vi "SCRAnalysis.vi"() -> ()   [LabVIEW 2013]
uses:
  <vilib>/Analysis/2dsp.llb/Decimate (single shot, DBL).vi
  <vilib>/Analysis/baseanly.llb/Real Dot Product.vi
  <vilib>/Utility/file.llb/Read From Spreadsheet File (DBL).vi
  <vilib>/Utility/file.llb/Read From Spreadsheet File (string).vi
  <vilib>/Utility/file.llb/Write To Spreadsheet File (DBL).vi
  <vilib>/measure/macond.llb/IIR Filter for 1 Chan.vi
  <vilib>/measure/maresamp.llb/Resample Waveform (single shot).vi
  <vilib>/Waveform/WDTFileIO.llb/Export Waveform To Spreadsheet File.vi
  <vilib>/Waveform/WDTFileIO.llb/ Write Waveform to File.vi
  <vilib>/Utility/file.llb/Write To Spreadsheet File (string).vi
  <vilib>/Analysis/NI_AALBase.lvlib
  <vilib>/Analysis/NI_AALPro.lvlib
  <vilib>/measure/NI_MAPro.lvlib
panel:
  out "subarray":string[][](array[string])
  out "raw data":dbl[][](array[numeric])
  in  "Tab Control":enum32{"Data Preprocessing", "SCR Analysis"}(tab)
  in  "Load Data":bool
  out "Cleaned Data":waveform(dbl)(graph)={"t0"=timestamp(0 s since 1904-01-01), "dt"=0.05, "Y"=[]}
  in  "Create Event Onset Files from Markers":bool caption="OK Button"
  in  "column containing SCR":i32=1
  in  "Start marker":string
  in  "Event markers of interest":string[](array[string])=["", "", "", "", "", "", "", "", "", "", "", ""]
  in  "Sample Rate (Hz)":dbl=20.0
  in  "Save Cleaned Data":bool
  in  "Apply New Settings":bool
  in  "New Sample Rate (Hz)":i32=25
  out "Raw Data":waveform(dbl)(graph)={"t0"=timestamp(0 s since 1904-01-01), "dt"=0.05, "Y"=[]}
  in  "Rank":i32=3 min=1
  in  "Filter?":bool
  in  "Median Filter?":bool
  in  "Resample Data":bool
  in  "IIR filter specifications":T1={"Topology"=enum."Butterworth", "Type"=enum."Bandpass", "Order"=1, "Lower Fc"=0.1, "Upper Fc"=5.0, "PB Ripple"=1.0, "SB Attenuation"=60.0} {"PB Ripple" format="%0.2f"; "SB Attenuation" format="%0.2f"; "Lower Fc" format="%0.2p"; "Upper Fc" format="%0.2p"}
  out "Event  Timepoints (in samples - first number in each row is number of events detected in the file)":i32[][](array[numeric])
  in  "column containing markers":i32=2
  out "start marker detected at row":i32
  in  "append text to start of each line":string
  in  "Timing file names":string
  in  "Timing file directory":path
  out "residual":dbl=0.00434139012463345
  in  "Event Offset (s)":dbl=-2.0
  in  "Save Coefficients":bool
  out "Basis Set":dbl[][](graph)
  out "Event-related responses":dbl[][](graph)
  out "All Regressors":dbl[][](graph)
  out "Data and Fitted Response":dbl[][](graph)
  in  "Number of Basis Functions":i32=8
  in  "Window Length (s)":dbl=12.0
  out "Coefficients (GLM parameter estimates)":dbl[](array[numeric])
  in  "recalculate":bool
  in  "Save Response Data":bool
  in  "decimating factor":i32=1
  in  "Basis Set":u16(ring)=1 items=["Fourier", "Tents", "Blocks"]
  in  "append to existing files?":bool
  # "Data Preprocessing"
  # "SCR Analysis"
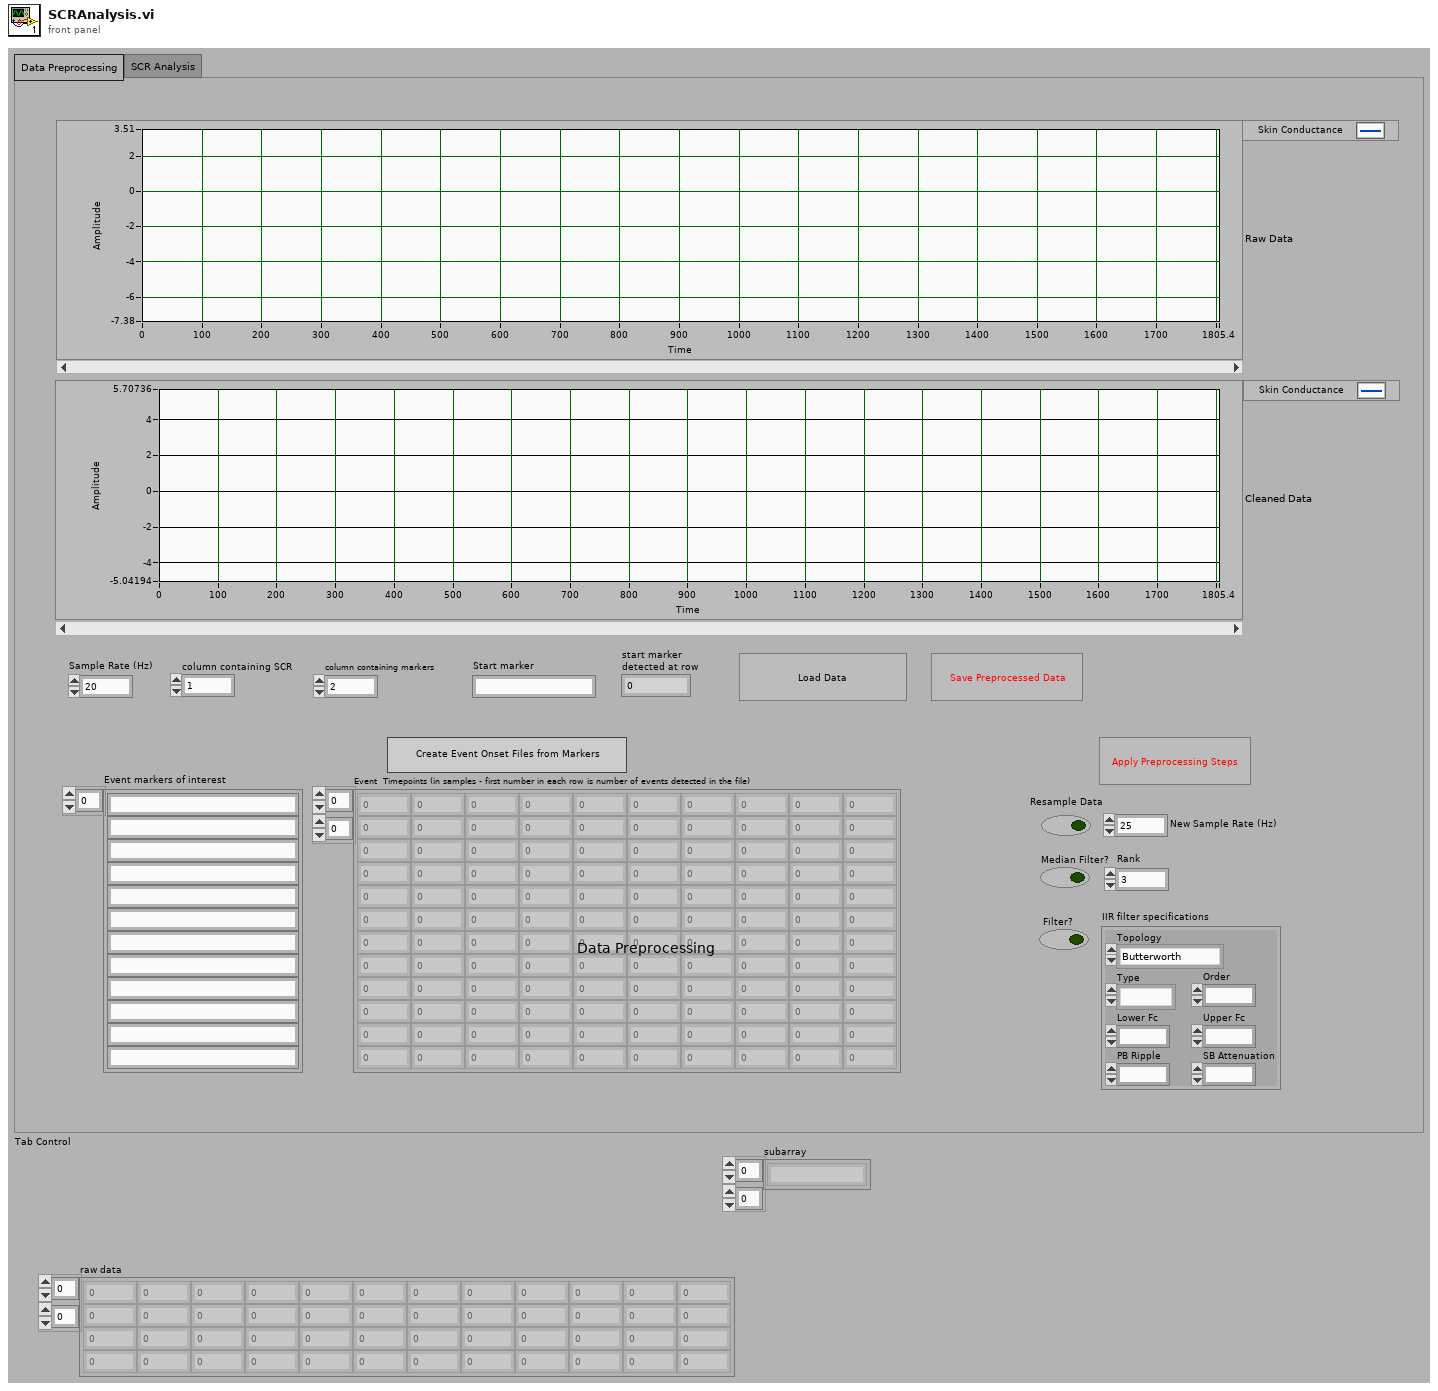
[diagram p1: front panel]
types:
  T1 = cluster{"Topology":enum16{"Off", "Butterworth", "Chebyshev", "Inverse Chebyshev", "Elliptic", "Bessel"}, "Type":enum16{"Lowpass", "Highpass", "Bandpass", "Bandstop"}, "Order":i32, "Lower Fc":dbl, "Upper Fc":dbl, "PB Ripple":dbl, "SB Attenuation":dbl}
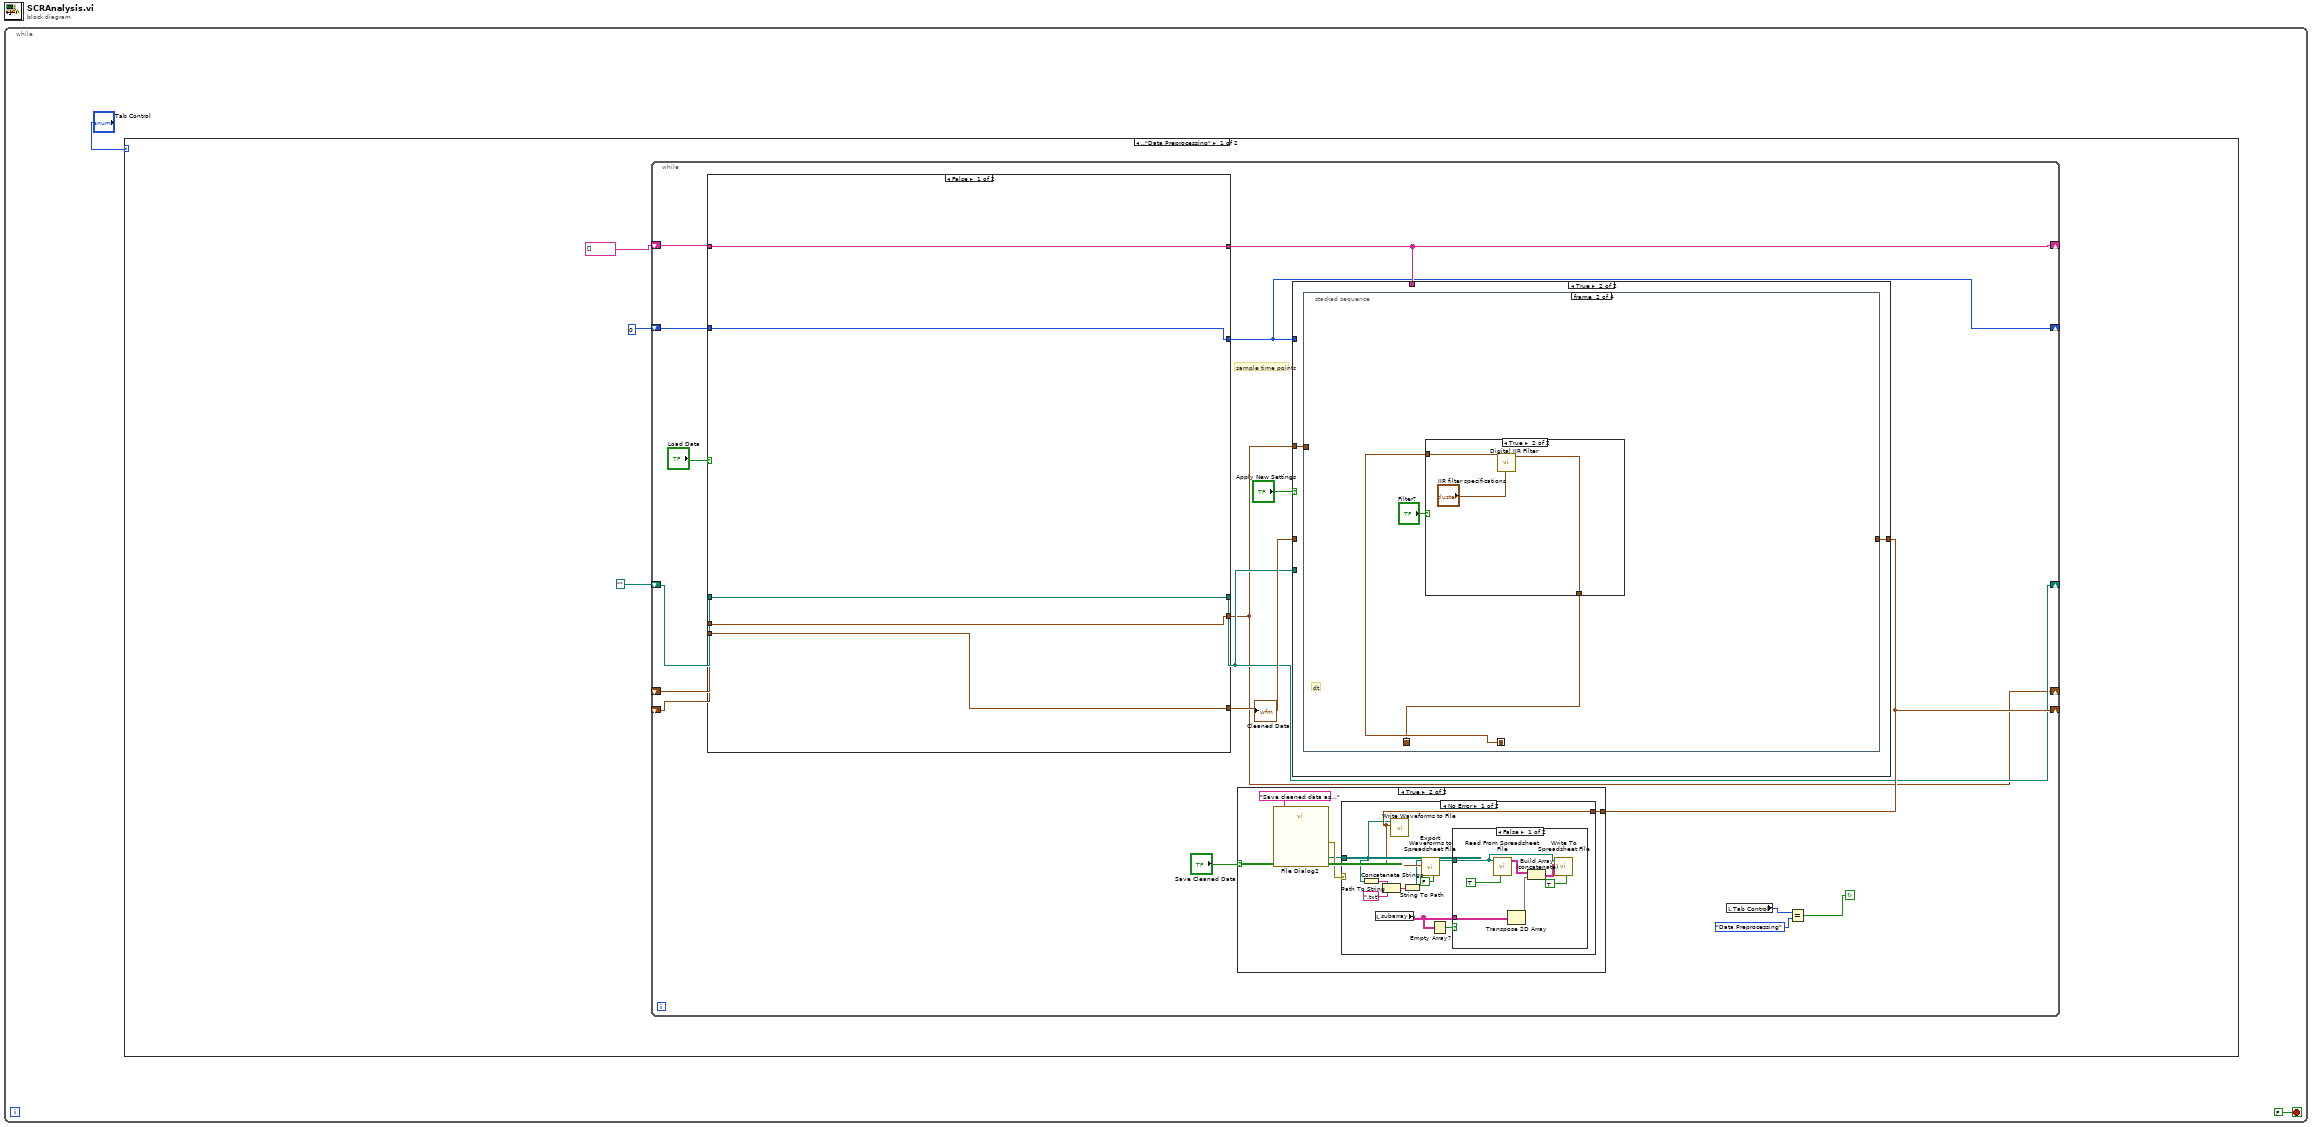
[diagram p0: block diagram]
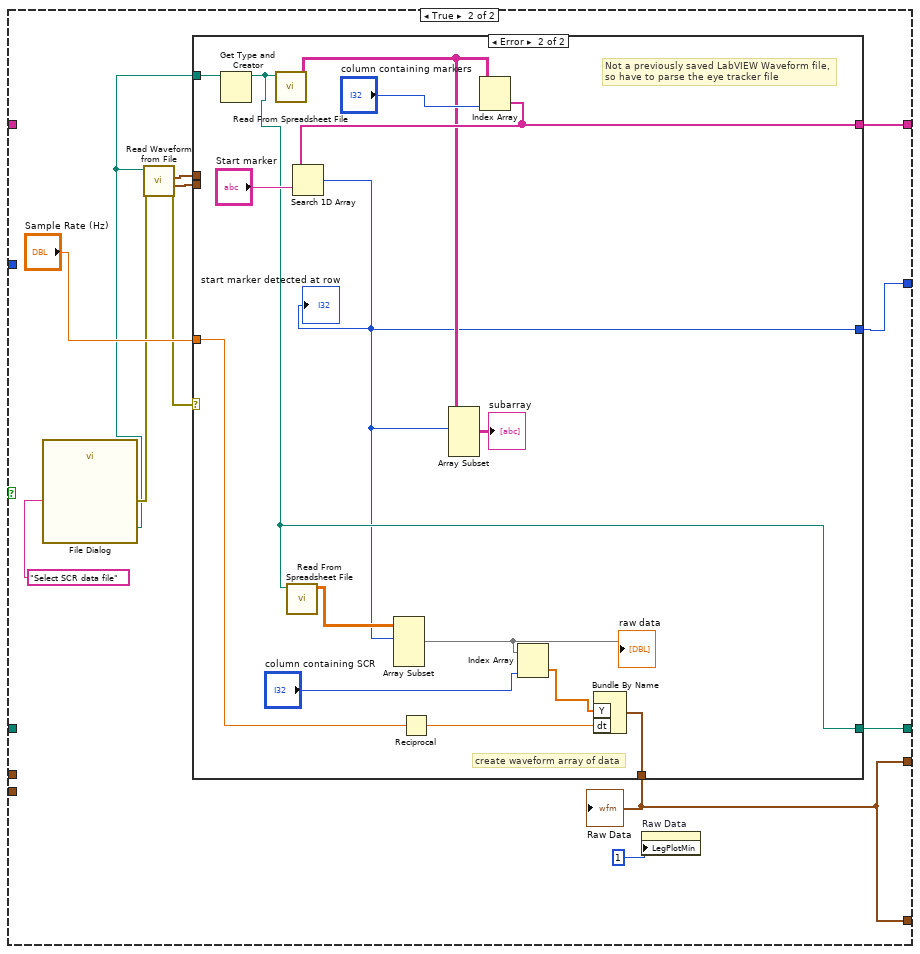
[diagram p2: hidden frame]
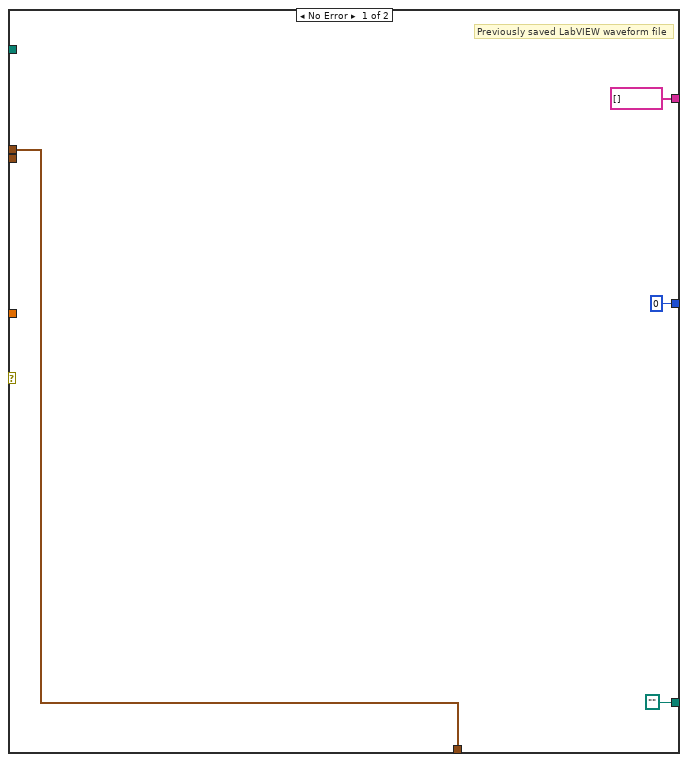
[diagram p3: hidden frame]
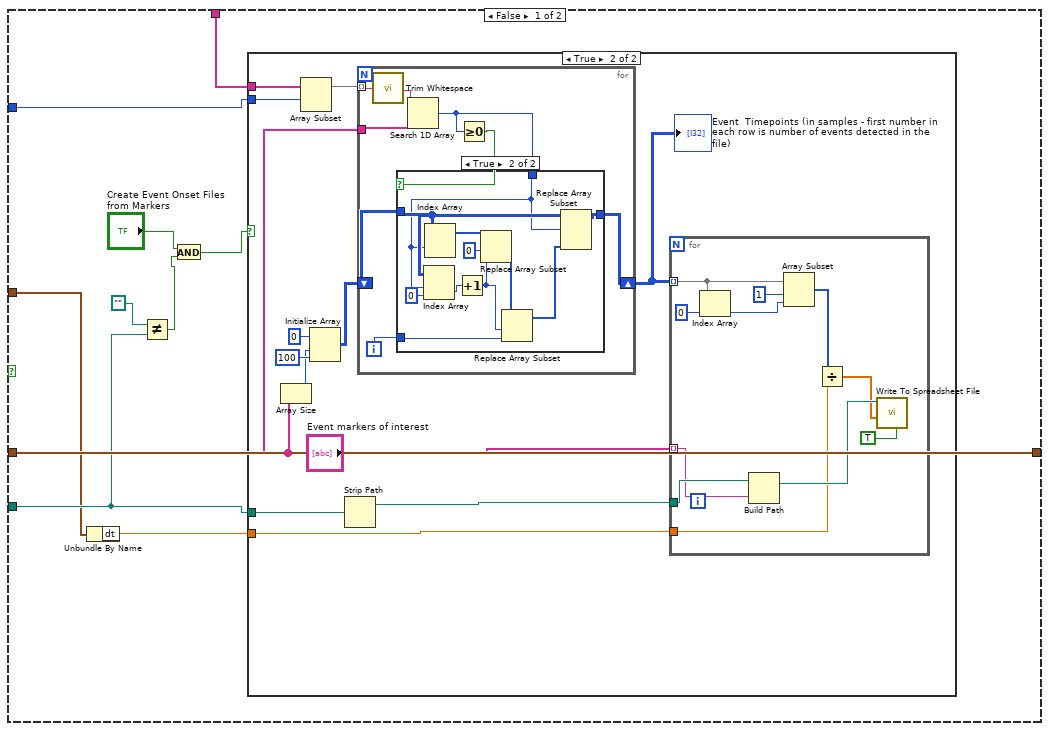
[diagram p7: hidden frame]
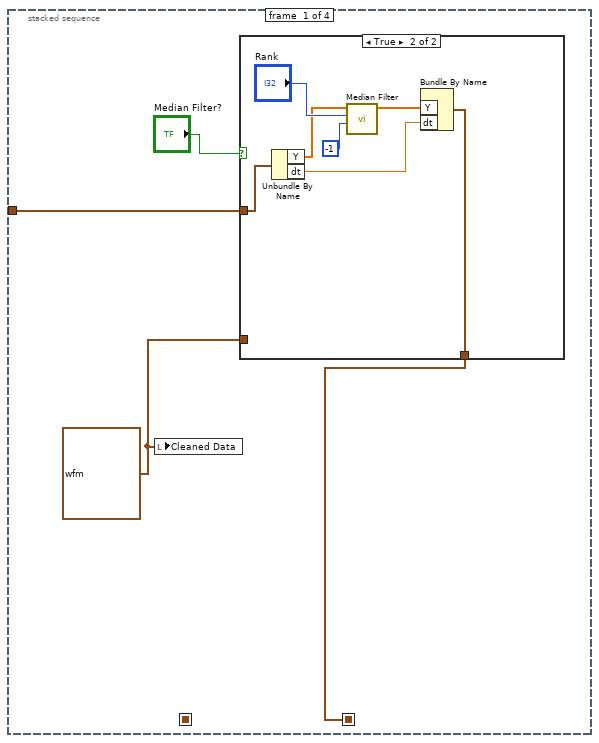
[diagram p10: hidden frame]
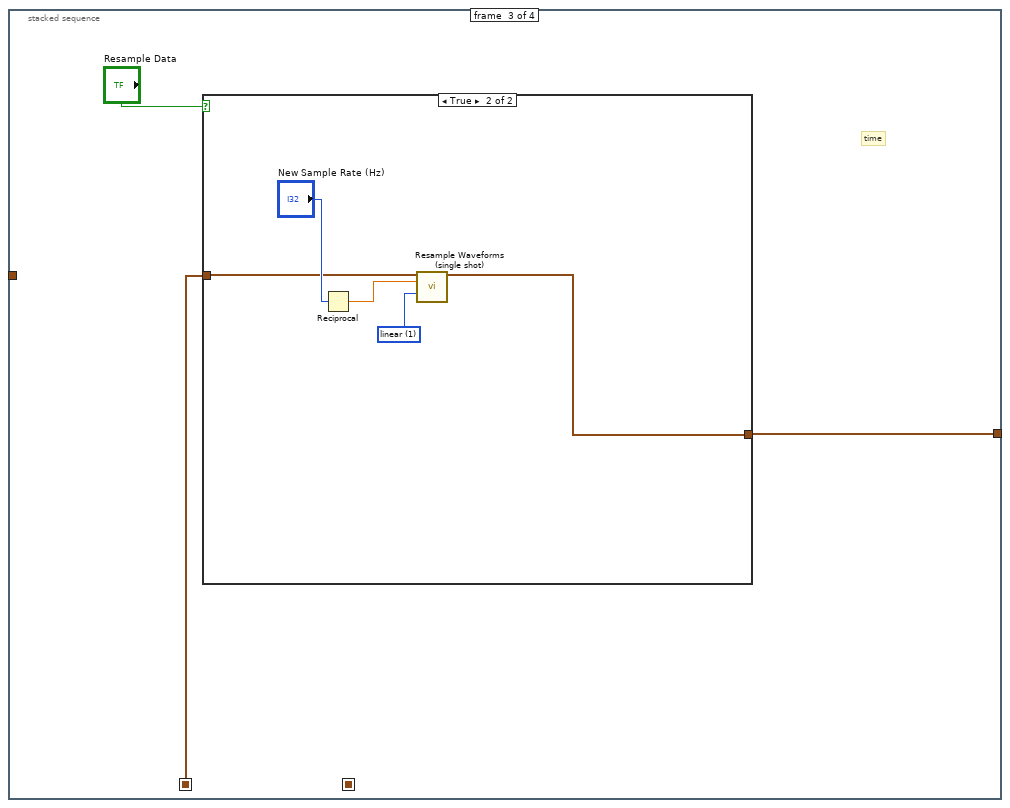
[diagram p13: hidden frame]
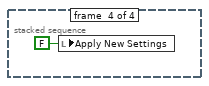
[diagram p15: hidden frame]
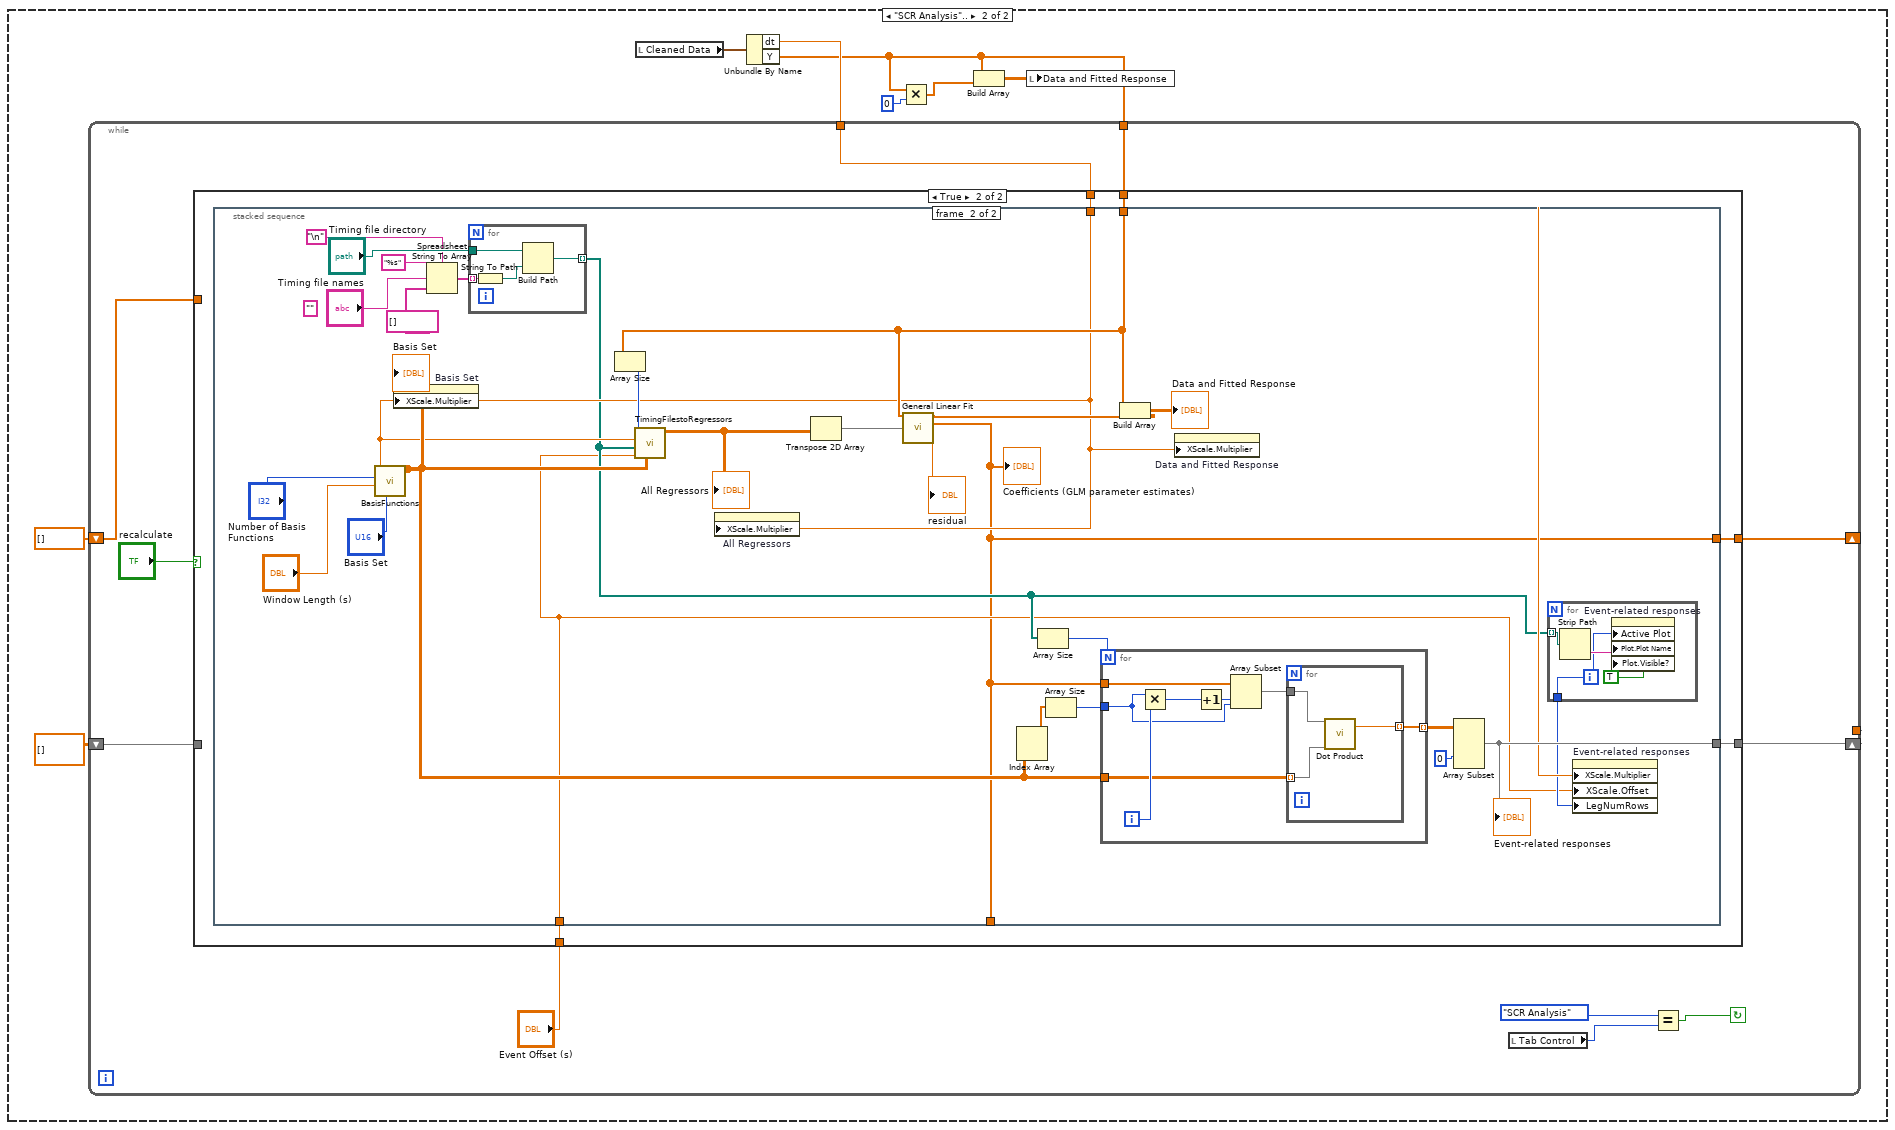
[diagram p16: hidden frame]
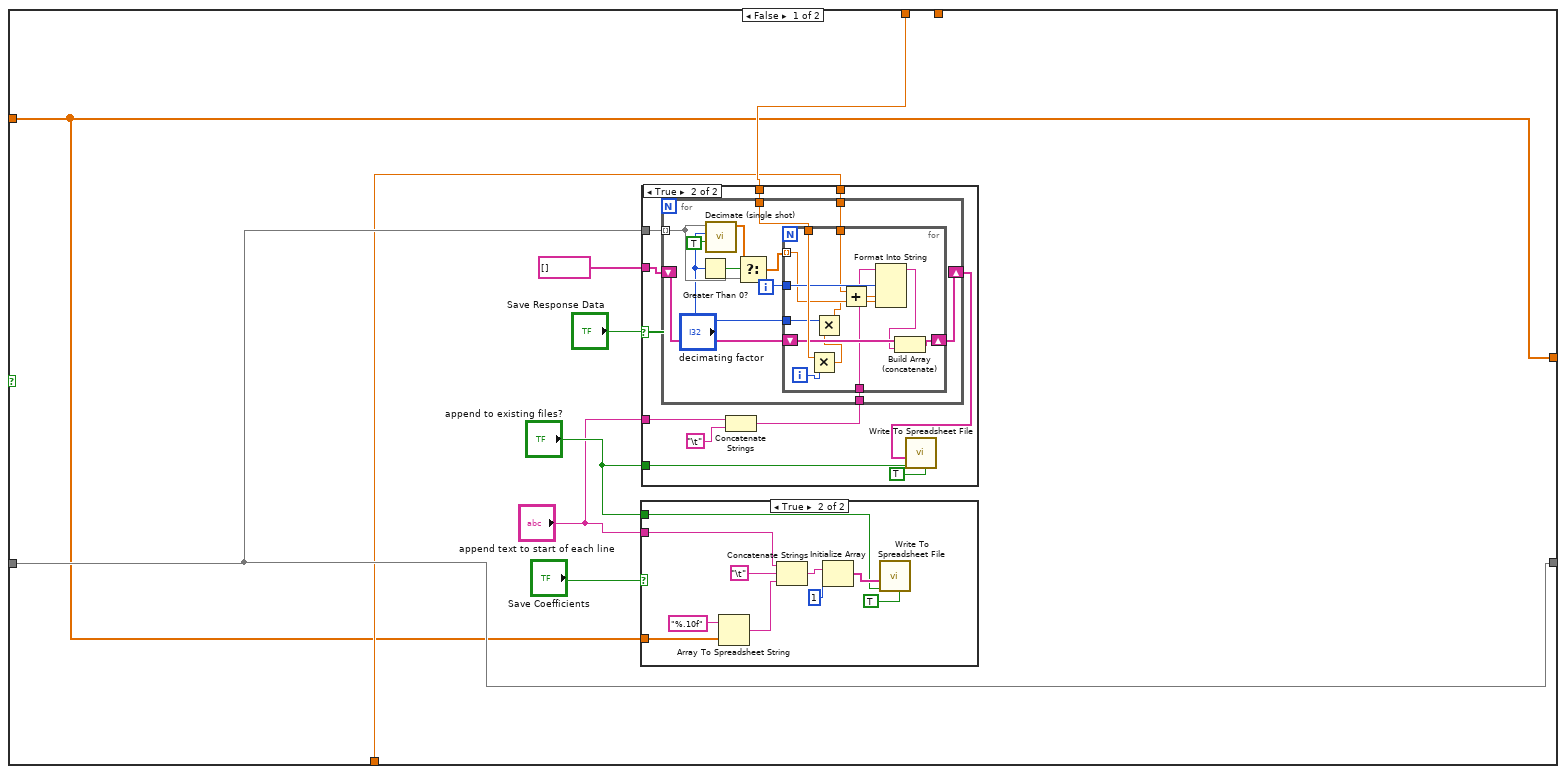
[diagram p17: hidden frame]
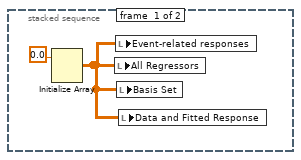
[diagram p20: hidden frame]
diagram:
  n1 = while {
    stop <- FALSE stop-if-true
    n2 = case shown="..\"Data Preprocessing\"" "Tab Control" {
      frame .."Data Preprocessing" {
        n3 = while {
          shift-right: [w20] -> _
          shift-left: _ -> [w15]
          shift-right: [w11] -> _
          shift-left: 0 ("index of element") -> [w18]
          shift-right: [w10] -> _
          shift-left: path "" ("path out") -> [w17]
          shift-right: [w9] -> _
          shift-left: _ -> [w16]
          shift-right: [w12] -> _
          shift-left: string[] [] ("all rows") -> [w13]
          stop <- w6 continue-if-true
          # "sample time points"
          n4 = case shown="False" "Load Data" {
            tunnel: [w25 w28] -> w9
            tunnel: [w27 w31] -> w11
            tunnel: [w23 w30] -> w12
            tunnel: w18 -> [w27 _]
            tunnel: [w26 w29] -> w10
            tunnel: w17 -> [w26 _]
            tunnel: w16 -> [w25 _]
            tunnel: [w24 w28] -> w14
            tunnel: w15 -> [w24 _]
            tunnel: w13 -> [w23 _]
            frame False {
            }
            frame True {
              n5 = call "File Dialog"("prompt"="Select SCR data file") -> ("selected path"=w35:path, "error out"=w36:errorcluster)  [unwired: 11 in, 2 out]
              n6 = call <vilib>:"Read Waveform from File.vi"("error in (no error)"=w36, "file path (dialog if empty)"=w35) -> ("error out"=w34:errorcluster, "all waveforms in record"=w32:waveform(dbl)[], "first waveform in record"=w33:waveform(dbl))  [unwired: 4 in, 1 out]
              n7 = case shown="Error" w34 {
                tunnel: [w43 w56] -> w28
                tunnel: w35 -> [_ w58]
                tunnel: w32 -> [_ _]
                tunnel: w33 -> [w43 _]
                tunnel: "Sample Rate (Hz)" -> [_ w48]
                tunnel: [path "" ("path out") w49] -> w29
                tunnel: [0 ("index of element") w45] -> w31
                tunnel: [string[] [] ("all rows") w47] -> w30
                frame No Error {
                  # "Previously saved LabVIEW waveform file"
                }
                frame Error {
                  # "Not a previously saved LabVIEW Waveform file,\nso have to parse the eye tracker file"
                  # "create waveform array of data"
                  n8 = Get Type and Creator(7:w58) -> (3:w49:path)  [unwired: 1 in, 3 out]
                  n9 = call-poly <vilib>:"Read From Spreadsheet File.vi"("file path (dialog if empty)"=w49) -> ("all rows"=w46:string[][])  [unwired: 6 in, 4 out]
                  n10 = call-poly <vilib>:"Read From Spreadsheet File.vi"("file path (dialog if empty)"=w49) -> ("all rows"=w53:dbl[][])  [unwired: 6 in, 4 out]
                  n11 = Reciprocal(x=w48) -> (1/x=w54:dbl)
                  n12 = Index Array(array=w46, index (col)="column containing markers") -> (element=w47:string[])  [unwired: 1 in]
                  n13 = Search 1D Array(1D array=w47, element="Start marker") -> (index of element=w45:i32)  [unwired: 1 in]
                  "start marker detected at row" <- w45
                  n14 = Array Subset(array=w53, index (row)=w45) -> (w52:dbl[][])  [unwired: 3 in]
                  "raw data" <- w52
                  n15 = Array Subset(array=w46, index (row)=w45) -> (→"subarray":string[][])  [unwired: 3 in]
                  n16 = Index Array(array=w52, index (col)="column containing SCR") -> (element=w55:dbl[])  [unwired: 1 in]
                  n17 = Bundle By Name("Y"=w55, "dt"=w54) -> (w56:waveform(dbl))  [unwired: 1 in]
                }
              }
              "Raw Data" <- w28
              n18 = property on="Raw Data" class="WFGraph (strict)"("LegPlotMin"=u32 1 ("Legend:Plot Minimum")) -> ()  [unwired: 2 in, 2 out]
            }
          }
          "Cleaned Data" <- w14
          n19 = case shown="True" "Apply New Settings" {
            tunnel: w9 -> [w81 w134]
            tunnel: [w89 w133] -> w20
            tunnel: w14 -> [w89 _]
            tunnel: w10 -> [w82 _]
            tunnel: w11 -> [w88 _]
            tunnel: w12 -> [w87 _]
            frame False {
              n20 = Unbundle By Name(w81) -> ("dt"=w80:dbl)
              n21 = Not Equal?(x=path "", y=w82) -> (x != y?=w85:bool)
              n22 = And(x="Create Event Onset Files from Markers", y=w85) -> (x .and. y?=w83:bool)
              n23 = case shown="True" w83 {
                tunnel: w82 -> [_ w100]
                tunnel: w80 -> [_ w98]
                tunnel: w87 -> [_ w97]
                tunnel: w88 -> [_ w95]
                frame False {
                }
                frame True {
                  n24 = Array Size(array="Event markers of interest") -> (size(s)=w93:i32)
                  n25 = Array Subset(array=w97, index=w95) -> (w96:string[])  [unwired: 1 in]
                  n26 = Initialize Array(0 ("element"), w93, 100 ("dimension size")) -> (w91:i32[][])
                  n27 = Strip Path(path=w100) -> (stripped path=w99:path)  [unwired: 1 out]
                  n28 = for {
                    tunnel: w96 -> [w113] mode=indexing
                    tunnel: "Event markers of interest" -> [w120]
                    shift-right: [w119] -> w101
                    shift-left: w91 -> [w118]
                    i -> [w115]
                    n29 = call <vilib>:"Trim Whitespace.vi"("string"=w113) -> ("trimmed string"=w114:string)  [unwired: 1 in]
                    n30 = Search 1D Array(1D array=w120, element=w114) -> (index of element=w117:i32)  [unwired: 1 in]
                    n31 = Greater Or Equal To 0?(x=w117) -> (x >= 0?=w116:bool)
                    n32 = case shown="True" w116 {
                      tunnel: [w121 w132] -> w119
                      tunnel: w118 -> [w121 w131]
                      tunnel: w117 -> [_ w130]
                      tunnel: w115 -> [_ w124]
                      frame False {
                      }
                      frame True {
                        n33 = Index Array(array=w131, index (row)=w130, index (col)=0 ("disabled index (col)")) -> (element=w128:i32)
                        n34 = Index Array(array=w131, index (row)=w130) -> (element=w126:i32[])  [unwired: 1 in]
                        n35 = Increment(x=w128) -> (x+1=w125:i32)
                        n36 = Replace Array Subset(array=w126, new element=w125, index=0) -> (w123:i32[])
                        n37 = Replace Array Subset(array=w123, new element=w124, index=w125) -> (w122:i32[])
                        n38 = Replace Array Subset(array=w131, new element=w122, index (row)=w130) -> (w132:i32[][])  [unwired: 1 in]
                      }
                    }
                  }
                  "Event  Timepoints (in samples - first number in each row is number of events detected in the file)" <- w101
                  n39 = for {
                    tunnel: "Event markers of interest" -> [w110] mode=indexing
                    tunnel: w101 -> [w103] mode=indexing
                    tunnel: w99 -> [w111]
                    tunnel: w98 -> [w108]
                    n40 = Index Array(array=w103, index=0) -> (element=w104:i32)
                    n41 = Build Path(base path=w111, name or relative path=w110) -> (appended path=w112:path)
                    n42 = Array Subset(array=w103, index=1, length=w104) -> (w102:i32[])
                    n43 = Divide(x=w102, y=w108) -> (x/y=w109:dbl[])
                    n44 = call-poly <vilib>:"Write To Spreadsheet File.vi"("transpose? (no:F)"=TRUE, "1D data"=w109, "file path (dialog if empty)"=w112) -> ()  [unwired: 5 in, 1 out]
                  }
                }
              }
            }
            frame True {
              n45 = stacked-sequence {
                seq-local: [w137 _ _ _] -> [_ w148 _ _]
                seq-local: [_ w147 _ _] -> [_ _ w154 _]
                tunnel: w134 -> [w136 _ _ _]
                tunnel: [_ _ w155 _] -> w133
                frame #0 {
                  w135 = waveform(dbl) {"t0"=timestamp(0 s since 1904-01-01), "dt"=1.0, "Y"=[]} ("signal out")
                  n46 = local write "Cleaned Data"(w135) -> ()
                  n47 = case shown="True" "Median Filter?" {
                    tunnel: w136 -> [w139 w142]
                    tunnel: [w139 w143] -> w137
                    tunnel: w135 -> [_ _]
                    frame False {
                    }
                    frame True {
                      n48 = Unbundle By Name(w142) -> ("Y"=w140:dbl[], "dt"=w141:dbl)
                      n49 = call <vilib>:"Median Filter.vi"("right rank"=-1, "left rank"="Rank", "X"=w140) -> ("Filtered X"=w145:dbl[])  [unwired: 7 in, 1 out]
                      n50 = Bundle By Name("Y"=w145, "dt"=w141) -> (w143:waveform(dbl))  [unwired: 1 in]
                    }
                  }
                }
                frame #1 {
                  # "dt"
                  n51 = case shown="True" "Filter?" {
                    tunnel: w148 -> [w150 w153]
                    tunnel: [w150 w151] -> w147
                    frame False {
                    }
                    frame True {
                      n52 = call-poly <vilib>:"Digital IIR Filter.vi"("IIR filter specifications"="IIR filter specifications", "signal in"=w153) -> ("signal out"=w151:waveform(dbl))  [unwired: 7 in, 2 out]
                    }
                  }
                }
                frame #2 {
                  # "time"
                  n53 = case shown="True" "Resample Data" {
                    tunnel: [w157 w159] -> w155
                    tunnel: w154 -> [w157 w161]
                    frame False {
                    }
                    frame True {
                      w160 = u16 1 items=["coerce", "linear", "spline", "FIR filter"] ("interpolation mode")
                      n54 = Reciprocal(x="New Sample Rate (Hz)") -> (1/x=w158:dbl)
                      n55 = call-poly <vilib>:"Resample Waveforms (single shot).vi"("waveform in"=w161, "dt"=w158, "interpolation mode"=w160) -> ("resampled waveform out"=w159:waveform(dbl))  [unwired: 9 in, 3 out]
                    }
                  }
                }
                frame #3 {
                  n56 = local write "Apply New Settings"(FALSE ("Apply New Settings")) -> ()
                }
              }
            }
          }
          n57 = case shown="True" "Save Cleaned Data" {
            tunnel: w20 -> [_ w60]
            frame False {
            }
            frame True {
              n58 = call "File Dialog2"("prompt"="Save cleaned data as...") -> ("selected path"=w59:path, "error out"=w61:errorcluster)  [unwired: 11 in, 2 out]
              n59 = case shown="No Error" w61 {
                tunnel: w60 -> [w72 _]
                tunnel: w59 -> [w71 _]
                frame No Error {
                  n60 = Path To String(path=w71) -> (string=w70:string)
                  n61 = local read "subarray"() -> (w63:string[][])
                  n62 = Concatenate Strings(w70, ".txt") -> (w68:string)
                  n63 = call-poly <vilib>:"Write Waveforms to File.vi"("waveform"=w72, "file path (dialog if empty)"=w71) -> ()  [unwired: 8 in, 2 out]
                  n64 = String To Path(string=w68) -> (path=w67:path)
                  n65 = call-poly <vilib>:"Export Waveforms to Spreadsheet File.vi"("header? (write header:T)"=FALSE, "waveform"=w72, "file path (dialog if empty)"=w67) -> ("new file path (Not A Path if cancelled)"=w65:path)  [unwired: 7 in, 1 out]
                  n66 = Empty Array?(array=w63) -> (empty?=w64:bool)
                  n67 = case shown="False" w64 {
                    tunnel: w65 -> [w76 _]
                    tunnel: w63 -> [w78 _]
                    frame False {
                      n68 = call-poly <vilib>:"Read From Spreadsheet File.vi"("transpose (no:F)"=TRUE, "file path (dialog if empty)"=w76) -> ("all rows"=w77:string[][])  [unwired: 5 in, 4 out]
                      n69 = Transpose 2D Array(2D array=w78) -> (transposed array=w73:string[][])
                      n70 = Build Array (concatenate)(w77, w73) -> (w75:string[][])
                      n71 = call-poly <vilib>:"Write To Spreadsheet File.vi"("transpose? (no:F)"=TRUE, "2D data"=w75, "file path (dialog if empty)"=w76) -> ()  [unwired: 5 in, 1 out]
                    }
                    frame True {
                    }
                  }
                }
                frame Error {
                }
              }
            }
          }
          n72 = local read "Tab Control"() -> (w7:enum32{"Data Preprocessing", "SCR Analysis"})
          n73 = Equal?(x=w7, y=enum32{"Data Preprocessing", "SCR Analysis"}."Data Preprocessing" ("Tab Control")) -> (x = y?=w6:bool)
        }
      }
      frame "SCR Analysis".. {
        n74 = local read "Cleaned Data"() -> (w167:waveform(dbl))
        n75 = Unbundle By Name(w167) -> ("dt"=w166:dbl, "Y"=w165:dbl[])
        n76 = while {
          tunnel: [w182] -> _
          shift-right: [w182] -> _
          shift-left: dbl[][] [] -> [w180]
          shift-right: [w178] -> _
          shift-left: dbl[] [] ("Coefficients") -> [w177]
          tunnel: w165 -> [w173]
          tunnel: w166 -> [w172]
          stop <- w176 continue-if-true
          n77 = case shown="True" "recalculate" {
            tunnel: [w186 w241] -> w182
            tunnel: w173 -> [_ w240]
            tunnel: w172 -> [w185 w239]
            tunnel: w180 -> [w186 _]
            tunnel: "Event Offset (s)" -> [w184 w238]
            tunnel: [w183 w237] -> w178
            tunnel: w177 -> [w183 _]
            frame False {
              n78 = case shown="True" "Save Coefficients" {
                tunnel: w183 -> [_ w200]
                tunnel: "append text to start of each line" -> [_ w198]
                tunnel: "append to existing files?" -> [_ w194]
                frame False {
                }
                frame True {
                  n79 = Array To Spreadsheet String(array=w200, 3:"%.10f" ("format (%.3f)")) -> (spreadsheet string=w199:string)  [unwired: 1 in]
                  n80 = Concatenate Strings(w198, "\t" ("string"), w199) -> (w195:string)
                  n81 = Initialize Array(w195, 1 ("dimension size")) -> (w196:string[])
                  n82 = call-poly <vilib>:"Write To Spreadsheet File.vi"("transpose? (no:F)"=TRUE, "append to file? (new file:F)"=w194, "1D data"=w196) -> ()  [unwired: 5 in, 1 out]
                }
              }
              n83 = case shown="True" "Save Response Data" {
                tunnel: w186 -> [_ w211]
                tunnel: w185 -> [_ w210]
                tunnel: "append text to start of each line" -> [_ w206]
                tunnel: "append to existing files?" -> [_ w207]
                tunnel: w184 -> [_ w203]
                tunnel: string[] [] -> [_ w202]
                frame False {
                }
                frame True {
                  n84 = Concatenate Strings(w206, "\t" ("string")) -> (w204:string)
                  n85 = for {
                    tunnel: w211 -> [w217] mode=indexing
                    shift-right: [w221] -> w209
                    shift-left: w202 -> [w220]
                    tunnel: w210 -> [w223]
                    tunnel: w204 -> [w213]
                    tunnel: w203 -> [w212]
                    i -> [w222]
                    n86 = Greater Than 0?(x="decimating factor") -> (x > 0?=w216:bool)
                    n87 = call-poly <vilib>:"Decimate (single shot).vi"("averaging"=TRUE, "decimating factor"="decimating factor", "X"=w217) -> ("Decimated Array"=w219:dbl[])  [unwired: 7 in, 1 out]
                    n88 = Select(t=w219, s=w216, f=w217) -> (s? t:f=w218:dbl[])
                    n89 = for {
                      tunnel: w218 -> [w229] mode=indexing
                      shift-right: [w234] -> w221
                      shift-left: w220 -> [w233]
                      tunnel: w223 -> [w235]
                      tunnel: w222 -> [w230]
                      tunnel: "decimating factor" -> [w231]
                      tunnel: w213 -> [w227]
                      tunnel: w212 -> [w224]
                      i -> [w236]
                      n90 = Multiply(x=w235, y=w236) -> (x*y=w232:dbl)
                      n91 = Multiply(x=w231, y=w232) -> (x*y=w225:dbl)
                      n92 = Add(x=w224, y=w225) -> (x+y=w226:dbl)
                      n93 = Format Into String(initial string=w227, w230, w226, w229) -> (resulting string=w228:string)  [unwired: 2 in, 1 out]
                      n94 = Build Array (concatenate)(w233, w228) -> (w234:string[])
                    }
                  }
                  n95 = call-poly <vilib>:"Write To Spreadsheet File.vi"("transpose? (no:F)"=TRUE, "append to file? (new file:F)"=w207, "1D data"=w209) -> ()  [unwired: 5 in, 1 out]
                }
              }
            }
            frame True {
              n96 = stacked-sequence {
                tunnel: [_ w264] -> w241
                tunnel: w240 -> [_ w256]
                tunnel: [_ w244] -> _
                tunnel: w239 -> [_ w248]
                tunnel: w238 -> [_ w245]
                tunnel: [_ w244] -> w237
                frame #0 {
                  n97 = Initialize Array(0.0 ("element")) -> (w242:dbl[][])  [unwired: 2 in]
                  n98 = local write "All Regressors"(w242) -> ()
                  n99 = local write "Event-related responses"(w242) -> ()
                  n100 = local write "Basis Set"(w242) -> ()
                  n101 = local write "Data and Fitted Response"(w242) -> ()
                }
                frame #1 {
                  (unwired) "" ("Timing file names")
                  n102 = call "BasisFunctions.vi"("Basis Set"="Basis Set", "Window Length (s)"="Window Length (s)", "Number of Basis Functions"="Number of Basis Functions", "dt"=w248) -> ("Array of Basis Functions"=w250:dbl[][])  [unwired: 7 in]
                  "Basis Set" <- w250
                  n103 = property on="Basis Set" class="WFGraph (strict)"("XScale.Multiplier"=w248) -> ()  [unwired: 2 in, 2 out]
                  n104 = Spreadsheet String To Array(delimiter (Tab)="\n", format string="%s", spreadsheet string="Timing file names", array type (2D Dbl)=string[] []) -> (array=w260:string[])
                  n105 = for {
                    tunnel: w260 -> [w279] mode=indexing
                    tunnel: "Timing file directory" -> [w278]
                    tunnel: [w276] -> w246 mode=indexing
                    n106 = String To Path(string=w279) -> (path=w277:path)
                    n107 = Build Path(base path=w278, name or relative path=w277) -> (appended path=w276:path)
                  }
                  n108 = Array Size(array=w256) -> (size(s)=w270:i32)
                  n109 = call "TimingFilestoRegressors.vi"("Uniform Event Offset (s)"=w245, "Array of Basis Functions"=w250, "Array of Timing Files"=w246, "dt"=w248, "Total Number of Samples"=w270) -> ("Array of Regressors"=w253:dbl[][])  [unwired: 6 in]
                  "All Regressors" <- w253
                  n110 = property on="All Regressors" class="WFGraph (strict)"("XScale.Multiplier"=w248) -> ()  [unwired: 2 in, 2 out]
                  n111 = Transpose 2D Array(2D array=w253) -> (transposed array=w271:dbl[][])
                  n112 = call <vilib>:"General Linear Fit.vi"("Y"=w256, "H"=w271) -> ("Best Fit"=w255:dbl[], "Coefficients"=w244:dbl[], "residue"=→"residual":dbl)  [unwired: 8 in, 3 out]
                  "Coefficients (GLM parameter estimates)" <- w244
                  n113 = Index Array(array=w250) -> (element=w249:dbl[])  [unwired: 2 in]
                  n114 = Array Size(array=w246) -> (size(s)=w252:i32)
                  n115 = Array Size(array=w249) -> (size(s)=w251:i32)
                  n116 = for {
                    N: w252 -> [_]
                    tunnel: w244 -> [w287]
                    tunnel: [w280] -> w268 mode=indexing
                    tunnel: w251 -> [w281]
                    tunnel: w250 -> [w284]
                    i -> [w285]
                    n117 = Multiply(x=w281, y=w285) -> (x*y=w282:i32)
                    n118 = Increment(x=w282) -> (x+1=w283:i32)
                    n119 = Array Subset(array=w287, index=w283, length=w281) -> (w286:dbl[])
                    n120 = for {
                      tunnel: w286 -> [w290]
                      tunnel: w284 -> [w289] mode=indexing
                      tunnel: [w288] -> w280 mode=indexing
                      n121 = call-poly <vilib>:"Dot Product.vi"("Y Vector"=w289, "X Vector"=w290) -> ("X * Y"=w288:dbl)  [unwired: 1 out]
                    }
                  }
                  n122 = Build Array(w256, w255) -> (→"Data and Fitted Response":dbl[][])
                  n123 = property on="Data and Fitted Response" class="WFGraph (strict)"("XScale.Multiplier"=w248) -> ()  [unwired: 2 in, 2 out]
                  n124 = Array Subset(array=w268, index (col)=0 ("index")) -> (w264:dbl[][])  [unwired: 3 in]
                  "Event-related responses" <- w264
                  n125 = for {
                    tunnel: w246 -> [w275] mode=indexing
                    tunnel: [w272] -> w247
                    i -> [w272]
                    n126 = Strip Path(path=w275) -> (name=w274:string)  [unwired: 1 out]
                    n127 = property on="Event-related responses" class="WFGraph (strict)"("Active Plot"=w272, "Plot.Plot Name"=w274, "Plot.Visible?"=TRUE ("Plot.Visible")) -> ()  [unwired: 2 in, 2 out]
                  }
                  n128 = property on="Event-related responses" class="WFGraph (strict)"("XScale.Multiplier"=w248, "XScale.Offset"=w245, "LegNumRows"=w247) -> ()  [unwired: 2 in, 2 out]
                }
              }
            }
          }
          n129 = local read "Tab Control"() -> (w174:enum32{"Data Preprocessing", "SCR Analysis"})
          n130 = Equal?(x=enum32{"Data Preprocessing", "SCR Analysis"}."SCR Analysis" ("Tab Control"), y=w174) -> (x = y?=w176:bool)
        }
        n131 = Multiply(x=w165, y=0) -> (x*y=w168:dbl[])
        n132 = Build Array(w165, w168) -> (w164:dbl[][])
        n133 = local write "Data and Fitted Response"(w164) -> ()
      }
    }
  }
